vi "Main.vi"() -> ()   [LabVIEW 2017]
uses:
  <vilib>/NI/Module Execution Interface/Engine Runtime/Execution States.ctl
  <vilib>/NI/Module Execution Interface/Engine Runtime/Fault.ctl
  <vilib>/NI/Tag Bus Module Framework/runtime/error classification.ctl
  <vilib>/NI/DCAF/addons/InstructionFrameworkSupport/FPGA_FGV_action.ctl
  <vilib>/NI/PowerElectronicsControl/BufferLogging/BufferConfig.ctl
  <vilib>/NI/Current Value Table/DataTypes/Double_Read.vi
  <vilib>/NI/Current Value Table/Type to Enum.vi
  <vilib>/NI/Current Value Table/DataTypes/Double_Type To Enum.vi
  Support/globals.vi
  <vilib>/FPGAPlugInAG/sbRIO-9607/niLvFpga_Open_sbRIO-9607.vi
  <vilib>/rvi/interface/common/dynamic/niFpgaDynamicAddResources.vi
  <vilib>/FPGAPlugInAG/Dynamic/niLvFpga_Reset_Dynamic.vi
  <vilib>/FPGAPlugInAG/Dynamic/niLvFpga_Run_Dynamic.vi
  <vilib>/NI/Current Value Table/FGVs/CVT Globals.vi
  <vilib>/NI/Current Value Table/FGVs/Tag Memory.vi
  <vilib>/NI/Current Value Table/Memory Block.vi
  <vilib>/NI/Current Value Table/DataTypes/Double_Memory Block.vi
  <vilib>/rvi/interface/nirviOpenFPGA/nirviOpenFPGA.xnode
  FPGA/Bitfiles/BaseApplication_FPGATarget_Firmware_UcBh6Emi2ng.lvbitx
  <vilib>/rvi/interface/nirviMethod/nirviMethod.xnode
  <vilib>/NI/Module Execution Interface/Engine Runtime/Engine Runtime Interface.lvclass
  <vilib>/NI/DCAF/Tag Editor Core/Framework Configuration Classes/target runtime/PL_Target Runtime.lvclass
  <vilib>/NI/PowerElectronicsControl/BufferLogging/BufferLogging.lvlib
  <vilib>/NI/DCAF/Modules/FPGAWaveform/execution/WaveformAcq runtime.lvclass
  <vilib>/NI/Current Value Table/Current Value Table.lvlib
  <vilib>/NI/Tag Bus Module Framework/runtime/TBM module execution interface.lvclass
panel:
  in  "Abort":bool
  in  "Tab Control":enum32{"Engine", "Snapshot"}(tab)
  out "Resource Usage":dbl[][](graph)
  out "engine status":T4(array[cluster])
  out "snapshot":waveform(sgl)[](graph)
  in  "Update Rate (sec)":dbl=5.0 caption="Time Target (s)"
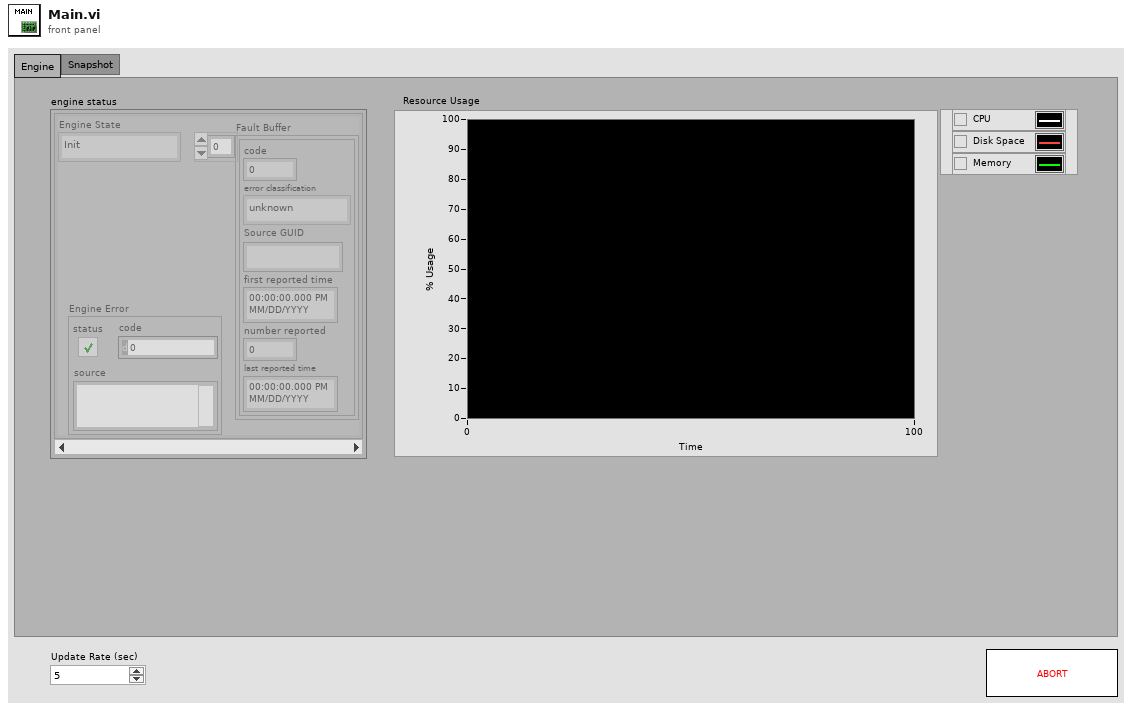
[diagram p1: front panel]
types:
  T1 = typedef "Engine Runtime Interface.lvclass/Execution States.ctl" = enum16{"Init", "Pre-Operational", "Safe-Operational", "Operational", "Stopped"}
  T2 = typedef "Engine Runtime Interface.lvclass/Fault.ctl" = cluster{"code":i32, "error classification":T3, "Source GUID":string, "first reported time":timestamp, "number reported":u32, "last reported time":timestamp}
  T3 = typedef "TBM module execution interface.lvclass/error classification.ctl" = enum16{"unknown", "none", "trivial", "recoverable", "critical"}
  T4 = cluster{"Engine State":T1, "Fault Buffer":T2[], "Engine Error":errorcluster}[]
  T5 = typedef "BufferLogging.lvlib/BufferConfig.ctl" = cluster{"Channels":string[], "pretriggerTime_sec":dbl, "posttriggerTime_sec":dbl, "BlockSizePerChannel":i32, "SampleRate_Hz":dbl, "decimation factor":i32, "logDirectory":string, "logPrefix":string, "max files":i32}
  T6 = typedef "FPGA_FGV_action.ctl" = enum16{"get FPGA", "set FPGA", "Close"}
  T7 = typedef "WaveformAcq runtime.lvclass/Export.ctl" = cluster{"instance":i32, "Queue Name":string, "StreamChannels":string[], "Sample rate":i32, "BufferSizePerChannel":i32, "SamplesPerRead":i32, "ReadTimeout":dbl}
  T8 = cluster{"Engine State":T1, "faults":T2[], "Engine Error":errorcluster}
  T9 = typedef "BufferLogging.lvlib/Buffers.ctl" = cluster{"Channels":string[], "PosttriggerBuffer":refnum<queue>, "PretriggerBuffer":refnum<queue>, "BlockSizePerChannel":i32, " logging semaphore":T10, "Log refnum":refnum<k34>, "snapshotBuffer":refnum<data-value>, "logDirectory":path, "logPrefix":string, "decimation factor":i32, "max files":i32, "SampleRate":dbl}
  T10 = typedef "Semaphore RefNum" = refnum<k1>
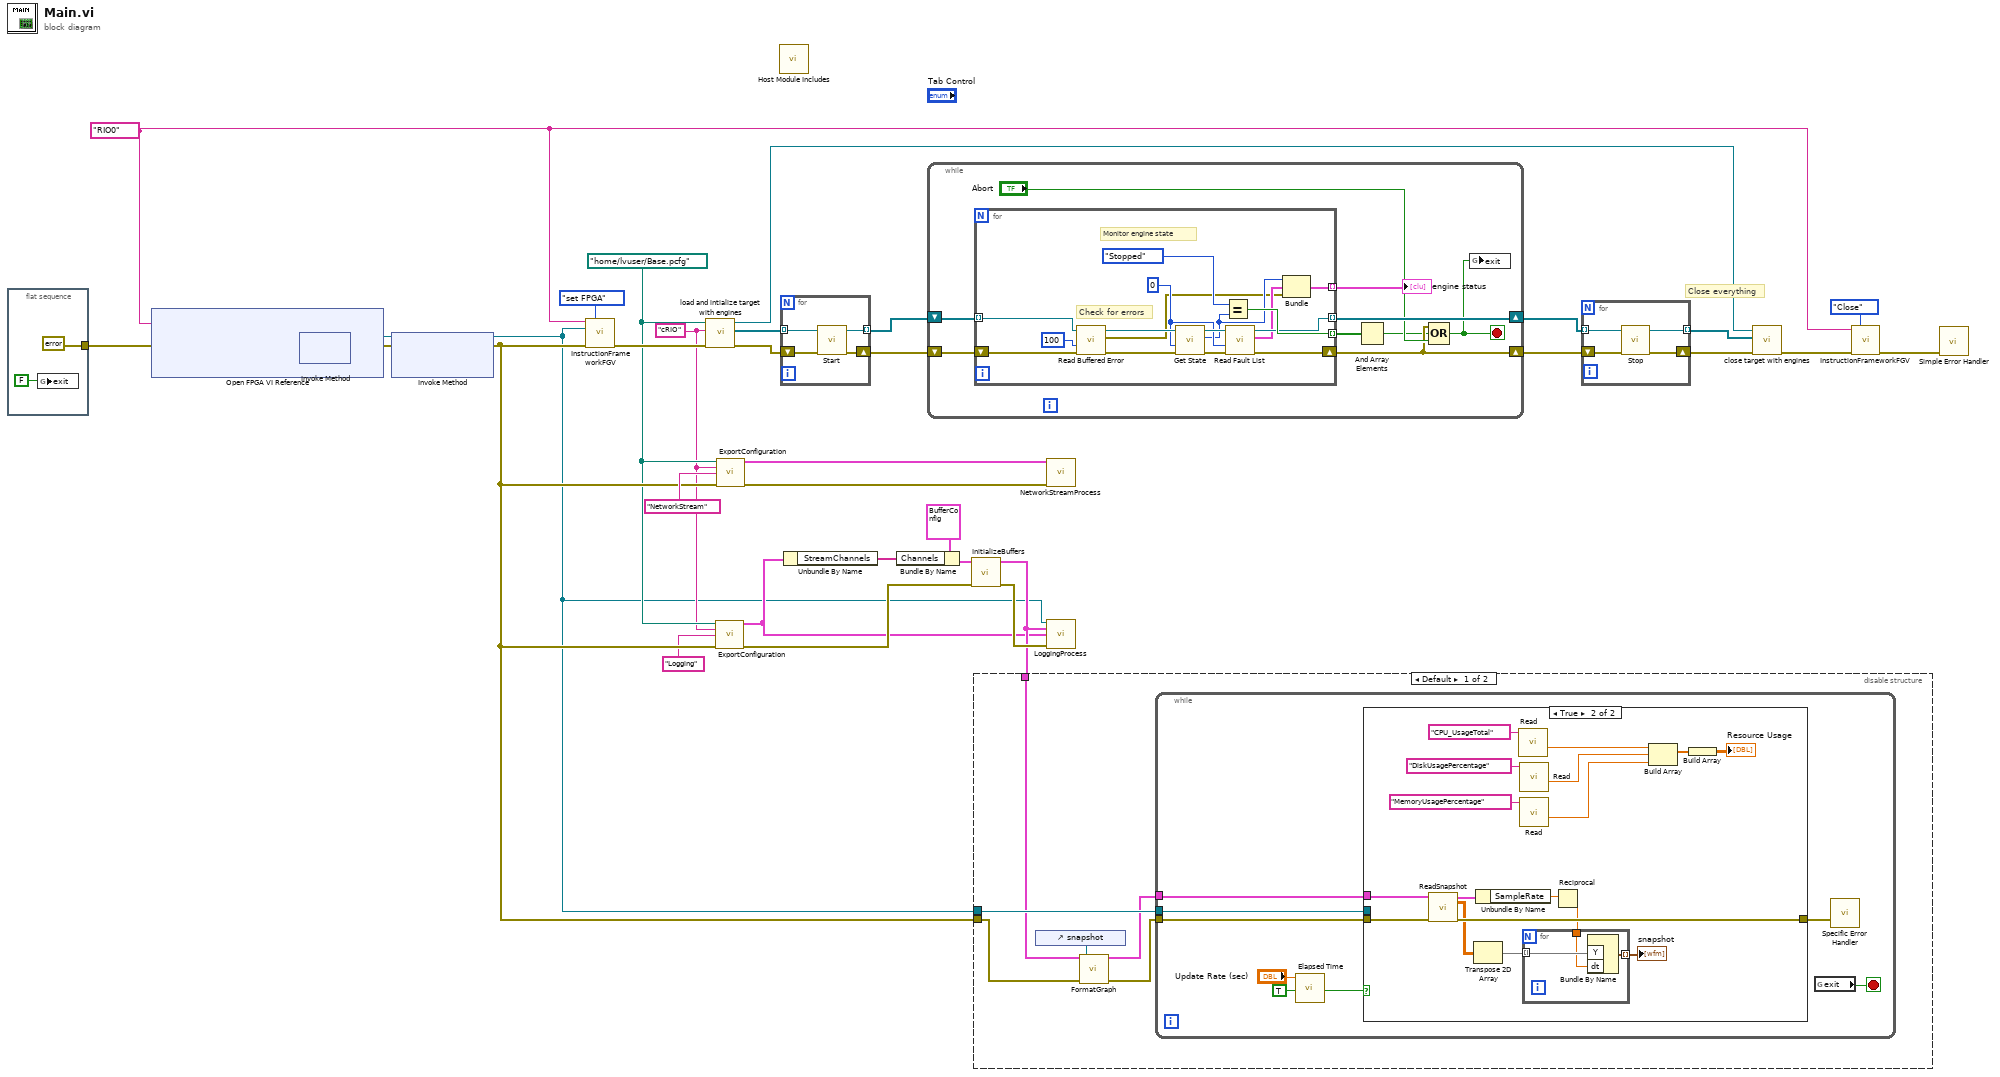
[diagram p0: block diagram]
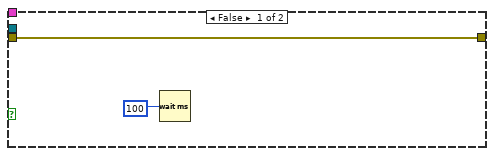
[diagram p2: hidden frame]
diagram:
  w2 = tag "RIO0" ("resource name")
  w8 = path "/home/lvuser/Base.pcfg" ("configuration file path")
  w7 = "cRIO" ("target alias")
  # "Close everything"
  n1 = flat-sequence {
    tunnel: [errorcluster {"status"=FALSE, "code"=0, "source"=""} ("error in")] -> w23
    frame #0 {
      n2 = global write "globals.vi" "exit"(FALSE ("exit")) -> ()
    }
  }
  n3 = xnode "Open FPGA VI Reference"("error in"=w23, "resource name"=w2) -> ("FPGA VI Reference Out"=w21:refnum<k20>, "error out"=w22:errorcluster)
  n4 = xnode "Invoke Method"("FPGA VI Reference In"=w21, "error in"=w22) -> ("FPGA VI Reference Out"=w20:refnum<k20>, "error out"=w19:errorcluster)
  n5 = xnode "Invoke Method"("FPGA VI Reference In"=w20, "error in"=w19) -> ("FPGA VI Reference Out"=w1:refnum<k20>, "error out"=w10:errorcluster)  [unwired: 1 in]
  n6 = call <vilib>:"InstructionFrameworkFGV.vi"("RIO resource"=w2, "Action"=FPGA_FGV_action."set FPGA", "bitfile to cache"=w1, "error in"=w10) -> ("error out"=w27:errorcluster)  [unwired: 9 in, 2 out]
  n7 = call <vilib>:"load and intialize target with engines.vi"("error in"=w27, "target alias"=w7, "file path"=w8) -> ("error out"=w32:errorcluster, "engine runtime interfaces"=w31:refnum<class "Engine Runtime Interface.lvclass">[], "target runtime"=w17:refnum<class "PL_Target Runtime.lvclass">)  [unwired: 6 in]
  n8 = call <vilib>:"ExportConfiguration.vi"("Path"=w8, "target alias"=w7, "Queue Name"="Logging" ("name (unnamed)"), "error in (no error)"=w10) -> ("ExportedConfiguration"=w4:T7, "error out"=w9:errorcluster)  [unwired: 10 in]
  n9 = call <vilib>:"ExportConfiguration.vi"("Path"=w8, "target alias"=w7, "Queue Name"="NetworkStream" ("name (unnamed)"), "error in (no error)"=w10) -> ("ExportedConfiguration"=w5:T7, "error out"=w11:errorcluster)  [unwired: 10 in]
  n10 = call "Host Module Includes.vi"() -> ()  [unwired: 12 in]
  n11 = for {
    tunnel: [w41] -> w35 mode=indexing
    tunnel: w31 -> [w38] mode=indexing
    shift-right: [w40] -> w28
    shift-left: w32 -> [w39]
    n12 = call-dynamic "Start.vi"("error in"=w39, "Engine Runtime Interface in"=w38) -> ("error out"=w40:errorcluster, "Engine Runtime Interface out"=w41:refnum<class "Engine Runtime Interface.lvclass">)  [unwired: 8 in]
  }
  n13 = Unbundle By Name(w4) -> ("StreamChannels"=w3:string[])
  n14 = Bundle By Name(cluster=T5 {"Channels"=["", "", "", "", "", "", "", "", "", "", "", "", "", "", "", "", "", "", "", "", "", "", "", "", "", "", "", "", "", "", "", "test"], "pretriggerTime_sec"=0.5, "posttriggerTime_sec"=0.5, "BlockSizePerChannel"=10000, "SampleRate_Hz"=100000.0, "decimation factor"=1, "logDirectory"="/home/lvuser/logs", "logPrefix"="log_", "max files"=5} ("BufferConfig"), "Channels"=w3) -> (w14:T5)
  n15 = while {
    shift-right: [w48] -> w34
    shift-left: w35 -> [w50]
    shift-right: [w46] -> w33
    shift-left: w28 -> [w49]
    stop <- w42 stop-if-true
    n16 = for {
      tunnel: w50 -> [w66] mode=indexing
      tunnel: [w57] -> w48 mode=indexing
      tunnel: [w61] -> w44 mode=indexing
      shift-right: [w56] -> w46
      shift-left: w49 -> [w65]
      tunnel: [w51] -> w45 mode=indexing
      w55 = 0 ("timeout (-1)")
      # "Monitor engine state"
      # "Check for errors"
      n17 = call-dynamic "Read Buffered Error.vi"("error in"=w65, "timeout in ms (0)"=100, "Engine Runtime Interface in"=w66) -> ("error out"=w63:errorcluster, "Engine Error"=w52:errorcluster, "Engine Runtime Interface out"=w64:refnum<class "Engine Runtime Interface.lvclass">)  [unwired: 6 in]
      n18 = call-dynamic "Get State.vi"("error in"=w63, "timeout (-1)"=w55, "Engine Runtime Interface in"=w64) -> ("error out"=w59:errorcluster, "Engine State"=w54:T1, "Engine Runtime Interface out"=w58:refnum<class "Engine Runtime Interface.lvclass">)  [unwired: 6 in]
      n19 = Equal?(x=Execution_States."Stopped" ("Engine State"), y=w54) -> (x = y?=w61:bool)
      n20 = call-dynamic "Read Fault List.vi"("error in"=w59, "timeout (-1)"=w55, "Engine Runtime Interface in"=w58) -> ("error out"=w56:errorcluster, "faults"=w53:T2[], "Engine Runtime Interface out"=w57:refnum<class "Engine Runtime Interface.lvclass">)  [unwired: 6 in]
      n21 = Bundle("Engine State"=w54, "faults"=w53, "Engine Error"=w52) -> (w51:T8)  [unwired: 1 in]
    }
    "engine status" <- w45
    n22 = And Array Elements(Boolean array=w44) -> (logical AND=w43:bool)
    n23 = Compound Arithmetic op=OR(w46, w43, "Abort") -> (w42:bool)
    n24 = global write "globals.vi" "exit"(w42) -> ()
  }
  n25 = call <vilib>:"InitializeBuffers.vi"("BufferConfig"=w14, "error in (no error)"=w9) -> ("Buffers"=w13:T9, "error out"=w16:errorcluster)  [unwired: 12 in]
  n26 = disable-structure shown="Default" {
    disable-tunnel: w1 -> [w72 _]
    disable-tunnel: w10 -> [w71 _]
    disable-tunnel: w13 -> [w69 _]
    frame condition #0 (active) {
      n27 = control-ref of="snapshot"() -> (w67:refnum<vi>)
      n28 = call "FormatGraph.vi"("Buffers in"=w69, "snapshotRef"=w67, "error in (no error)"=w71) -> ("Buffers out"=w68:T9, "error out"=w70:errorcluster)  [unwired: 11 in]
      n29 = while {
        tunnel: w72 -> [w74]
        tunnel: w70 -> [w73]
        tunnel: w68 -> [w75]
        stop <- w80 stop-if-true
        n30 = call "Elapsed Time"("Time Target (s)"="Update Rate (sec)", "Auto Reset"=TRUE) -> ("Time has Elapsed"=w78:bool)  [unwired: 10 in, 7 out]
        n31 = case shown="True" w78 {
          tunnel: w73 -> [w82 w99]
          tunnel: w74 -> [_ _]
          tunnel: [w82 w98] -> w76
          tunnel: w75 -> [_ w97]
          frame False {
            n32 = Wait (ms)(milliseconds to wait=u32 100) -> ()  [unwired: 1 out]
          }
          frame True {
            n33 = call <vilib>:"ReadSnapshot.vi"("Buffers in"=w97, "error in (no error)"=w99) -> ("Buffers out"=w93:T9, "snapshot"=w96:sgl[][], "error out"=w98:errorcluster)  [unwired: 11 in]
            n34 = Transpose 2D Array(2D array=w96) -> (transposed array=w95:sgl[][])
            n35 = Unbundle By Name(w93) -> ("SampleRate"=w92:dbl)
            n36 = call-poly <vilib>:"Read.vi"("Tag Name"="CPU_UsageTotal") -> ("Value"=w87:dbl)  [unwired: 9 in, 1 out]
            n37 = call-poly <vilib>:"Read.vi"("Tag Name"="DiskUsagePercentage") -> ("Value"=w84:dbl)  [unwired: 9 in, 1 out]
            n38 = call-poly <vilib>:"Read.vi"("Tag Name"="MemoryUsagePercentage") -> ("Value"=w83:dbl)  [unwired: 9 in, 1 out]
            n39 = Reciprocal(x=w92) -> (1/x=w91:dbl)
            n40 = for {
              tunnel: w95 -> [w102] mode=indexing
              tunnel: [w101] -> w94 mode=indexing
              tunnel: w91 -> [w100]
              n41 = Bundle By Name("Y"=w102, "dt"=w100) -> (w101:waveform(sgl))  [unwired: 1 in]
            }
            "snapshot" <- w94
            n42 = Build Array(w87, w84, w83) -> (w86:dbl[])
            n43 = Build Array(w86) -> (→"Resource Usage":dbl[][])
          }
        }
        n44 = global read "globals.vi" "exit"() -> (w80:bool)
        n45 = call "Specific Error Handler"("Error to Check"=w76) -> ()  [unwired: 11 in, 4 out]
      }
    }
    frame condition #1 {
    }
  }
  n46 = call "NetworkStreamProcess.vi"("WaveformConfiguration"=w5, "error in (no error)"=w11) -> ()  [unwired: 14 in]
  n47 = call "LoggingProcess.vi"("FPGA Interface"=w1, "Buffers"=w13, "WaveformConfiguration"=w4, "error in (no error)"=w16) -> ()  [unwired: 12 in]
  n48 = for {
    tunnel: w34 -> [w106] mode=indexing
    shift-right: [w103] -> w29
    shift-left: w33 -> [w105]
    tunnel: [w104] -> w30 mode=indexing
    n49 = call-dynamic "Stop.vi"("error in"=w105, "Engine Runtime Interface in"=w106) -> ("error out"=w103:errorcluster, "Engine Runtime Interface out"=w104:refnum<class "Engine Runtime Interface.lvclass">)  [unwired: 8 in]
  }
  n50 = call <vilib>:"close target with engines.vi"("error in"=w29, "Engine Runtime Interfaces"=w30, "Target Runtime"=w17) -> ("error out"=w24:errorcluster)  [unwired: 8 in]
  n51 = call <vilib>:"InstructionFrameworkFGV.vi"("RIO resource"=w2, "Action"=FPGA_FGV_action."Close", "error in"=w24) -> ("error out"=w18:errorcluster)  [unwired: 10 in, 2 out]
  n52 = call <vilib>:"Simple Error Handler.vi"("error in (no error)"=w18) -> ()  [unwired: 4 in, 5 out]
